vi "Write and Read Multiple Holding Registers.vi"(4 "read count":u16, 6 "read starting address":u16, 7 "unit ID":u8, 8 "error in":errorcluster, 9 "write values":u16[](array[numeric]), 10 "write starting address":u16, 11 "Modbus instance in":refnum<class "Modbus Slave.lvclass">) -> (0 "error out":errorcluster, 1 "read values":u16[](array[numeric]), 3 "Modbus instance out":refnum<class "Modbus Slave.lvclass">)   [LabVIEW 2013, in "Modbus Library - Advance.lvlib" / "Modbus Slave.lvclass"]
doc: "Writes and reads the values of multiple register values in series. The <b>write values</b> are inserted starting at <b>write starting address</b> and the returned <b>read values</b> consists of <b>read count</b> holding registers starting at <b>read starting address</b>."
uses:
  Modbus Slave.lvclass
  Modbus Slave.lvclass/Modbus Slave.ctl
  Standard Data Model/Standard Data Model.lvclass
  Super Data Model/Super Data Model.lvclass
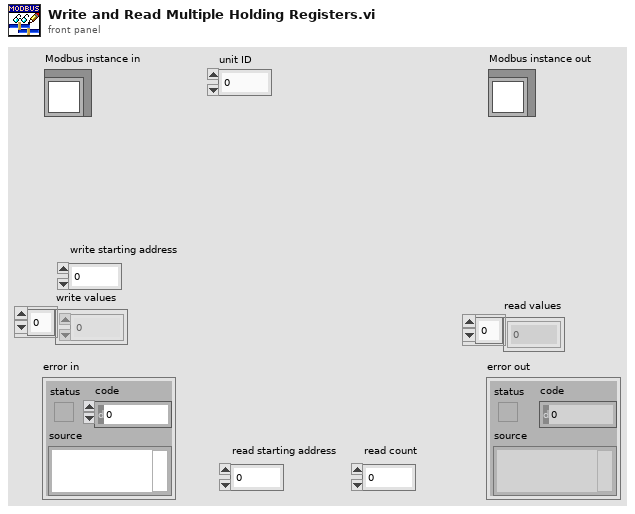
[diagram p1: front panel]
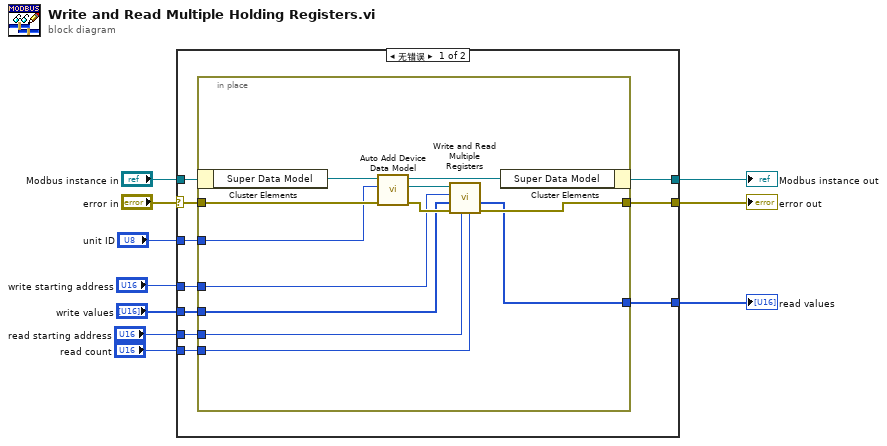
[diagram p0: block diagram]
diagram:
  n1 = case shown="无错误" "error in" {
    selector: "error in" -> [w20 w34]
    tunnel: "unit ID" -> [w19 _]
    tunnel: "Modbus instance in" -> [w18 w33]
    tunnel: [w17 w33] -> w3
    tunnel: [w16 w34] -> w1
    tunnel: "write starting address" -> [w15 _]
    tunnel: "write values" -> [w14 _]
    tunnel: "read starting address" -> [w13 _]
    tunnel: "read count" -> [w12 _]
    tunnel: [w11 _] -> w2
    frame No Error {
      n2 = in-place {
        in-place-border: w20 -> [w30]
        in-place-border: [w32] -> w16
        in-place-border: w19 -> [w29]
        in-place-border: w15 -> [w26]
        in-place-border: w14 -> [w25]
        in-place-border: w13 -> [w24]
        in-place-border: w12 -> [w23]
        in-place-border: [w22] -> w11
        n3 = in-place-cluster #1(w18) -> ("Super Data Model"=w31:refnum<class "Super Data Model.lvclass">)
        n4 = call "Auto Add Device Data Model.vi"("error in"=w30, "unit ID"=w29, "Super Data Model in"=w31) -> ("error out"=w27:errorcluster, "device data model"=w21:refnum<class "Standard Data Model.lvclass">, "Super Data Model out"=w28:refnum<class "Super Data Model.lvclass">)  [unwired: 6 in]
        n5 = call-dynamic "Write and Read Multiple Registers.vi"("read count"=w23, "read starting address"=w24, "error in"=w27, "write values"=w25, "write starting address"=w26, "device data model in"=w21) -> ("error out"=w32:errorcluster, "read values"=w22:u16[])  [unwired: 3 in, 1 out]
        n6 = in-place-cluster #1("Super Data Model"=w28) -> (w17:refnum<class "Modbus Slave.lvclass">)
      }
    }
    frame Error {
    }
  }
  "error out" <- w1
  "Modbus instance out" <- w3
  "read values" <- w2
